vi "Lockin.DAQ.Simulate Waveguide.vi"(8 "error in (no error)":errorcluster, 9 "Waveguide Cluster":T1={"Vsource Index"=0, "Vsg Index"=1, "V+"=0, "V-"=0}, 10 "AO []":waveform(dbl)[](array[waveform]), 11 "Lockin.DAQ in":refnum<class "Lockin.DAQ.lvclass">) -> (0 "error out":errorcluster, 2 "AI []":waveform(dbl)[](array[waveform]), 3 "Lockin.DAQ out":refnum<class "Lockin.DAQ.lvclass">)   [LabVIEW 2019, in "Lockin.DAQ.lvclass"]
uses:
  Lockin.DAQ.lvclass
  Waveguide Model/Waveguide Model--Cluster.ctl
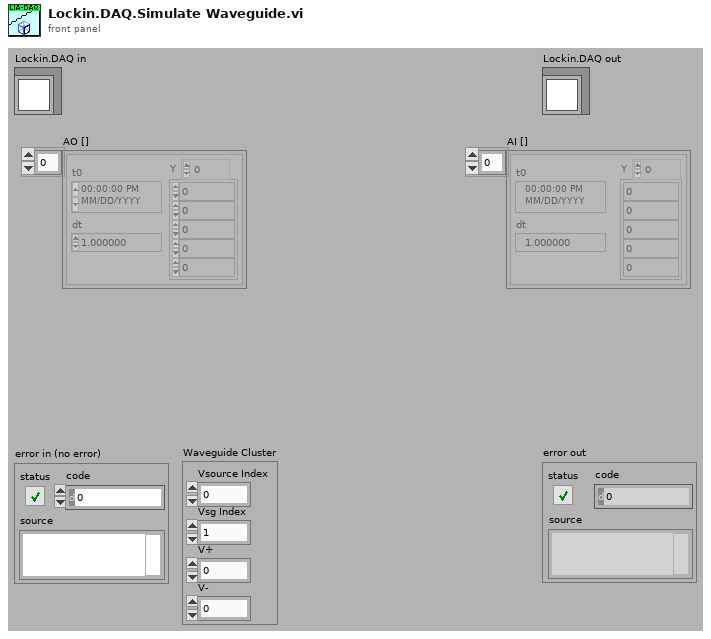
[diagram p1: front panel]
types:
  T1 = typedef "Lockin.DAQ.lvclass/Waveguide Model--Cluster.ctl" = cluster{"Vsource Index":i32, "Vsg Index":i32, "V+":i32, "V-":i32}
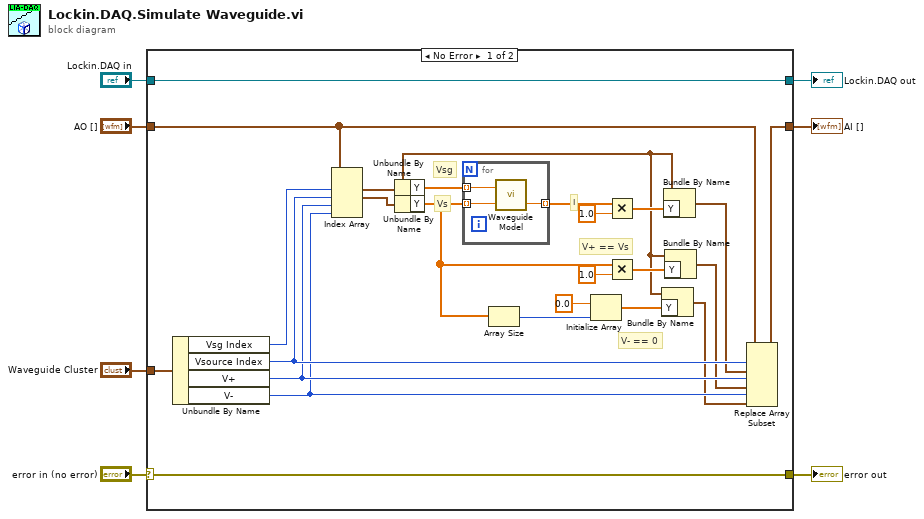
[diagram p0: block diagram]
diagram:
  n1 = case shown="No Error" "error in (no error)" {
    selector: "error in (no error)" -> [w9 w35]
    tunnel: "Waveguide Cluster" -> [w28 _]
    tunnel: [w25 w36] -> w6
    tunnel: [w9 w35] -> w4
    tunnel: [w8 w37] -> w3
    tunnel: "Lockin.DAQ in" -> [w8 w37]
    tunnel: "AO []" -> [w26 w36]
    frame No Error {
      # "V- == 0"
      # "V+ == Vs"
      # "I"
      # "Vs"
      # "Vsg"
      n2 = Unbundle By Name(w28) -> ("Vsg Index"=w24:i32, "Vsource Index"=w22:i32, "V+"=w21:i32, "V-"=w20:i32)
      n3 = Index Array(array=w26, index #1=w24, index #2=w22, index #3=w21, index #4=w20) -> (element #1=w11:waveform(dbl), element #2=w23:waveform(dbl))  [unwired: 2 out]
      n4 = Unbundle By Name(w11) -> ("Y"=w27:dbl[])
      n5 = Unbundle By Name(w23) -> ("Y"=w15:dbl[])
      n6 = for {
        tunnel: w15 -> [w34] mode=indexing
        tunnel: w27 -> [w33] mode=indexing
        tunnel: [w32] -> w30 mode=indexing
        n7 = call "Waveguide Model.vi"("Vs (V)"=w34, "Vsg (V)"=w33) -> ("I[Vsg] (A)"=w32:dbl)  [unwired: 1 out]
      }
      n8 = Array Size(array=w15) -> (size(s)=w14:i32)
      n9 = Initialize Array(0.0 ("y"), w14) -> (w12:dbl[])
      n10 = Multiply(x=w30, y=1.0) -> (x*y=w29:dbl[])
      n11 = Multiply(x=w15, y=1.0) -> (x*y=w17:dbl[])
      n12 = Bundle By Name(cluster=w11, "Y"=w12) -> (w10:waveform(dbl))
      n13 = Bundle By Name(cluster=w11, "Y"=w29) -> (w19:waveform(dbl))
      n14 = Bundle By Name(cluster=w11, "Y"=w17) -> (w16:waveform(dbl))
      n15 = Replace Array Subset(array=w26, new element #1=w19, index #1=w22, new element #2=w16, index #2=w21, new element #3=w10, index #3=w20) -> (w25:waveform(dbl)[])
    }
    frame Error {
    }
  }
  "error out" <- w4
  "Lockin.DAQ out" <- w3
  "AI []" <- w6
